vi "Read_Character.vi"() -> ()   [LabVIEW 2019]
uses:
  <vilib>/Utility/error.llb/DialogType.ctl
panel:
  out "Test From File:":string
  in  "File Path:":path
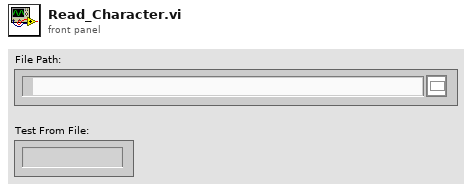
[diagram p1: front panel]
types:
  T1 = typedef "DialogType.ctl" = u16
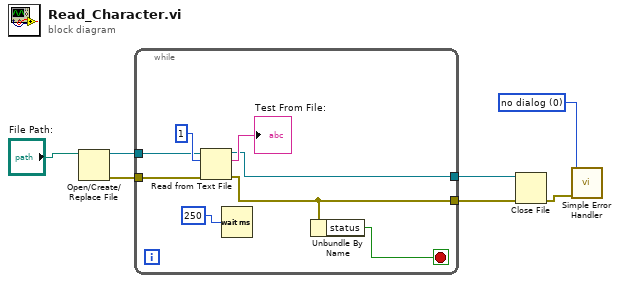
[diagram p0: block diagram]
diagram:
  w1 = T1 0 items=["no dialog", "OK message", "continue or stop message", "OK message + warnings", "continue/stop + warnings"] ("type of dialog (OK msg:1)")
  n1 = Open/Create/Replace File(file path (use dialog)="File Path:") -> (refnum out=w6:refnum<file>, error out=w4:errorcluster)  [unwired: 5 in, 1 out]
  n2 = while {
    tunnel: w6 -> [w13]
    tunnel: [w12] -> w5
    tunnel: w4 -> [w10]
    tunnel: [w9] -> w3
    stop <- w8 stop-if-true
    n3 = Read from Text File(file (use dialog)=w13, count=1, error in=w10) -> (refnum out=w12:refnum<file>, text=→"Test From File:":string, error out=w9:errorcluster)  [unwired: 1 in, 1 out]
    n4 = Wait (ms)(milliseconds to wait=u32 250) -> ()  [unwired: 1 out]
    n5 = Unbundle By Name(w9) -> ("status"=w8:bool)
  }
  n6 = Close File(refnum=w5, error in=w3) -> (error out=w2:errorcluster)  [unwired: 1 out]
  n7 = call <vilib>:"Simple Error Handler.vi"("type of dialog (OK msg:1)"=w1, "error in (no error)"=w2) -> ()  [unwired: 3 in, 5 out]
